vi "slider_inlet.vi"(10 "dq/dt (Flow in rate)\n[m³/s]":dbl, 11 "Slide in":refnum<vi>) -> ()   [LabVIEW 2020]
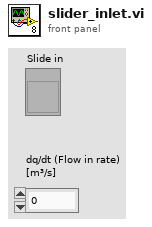
[diagram p1: front panel]
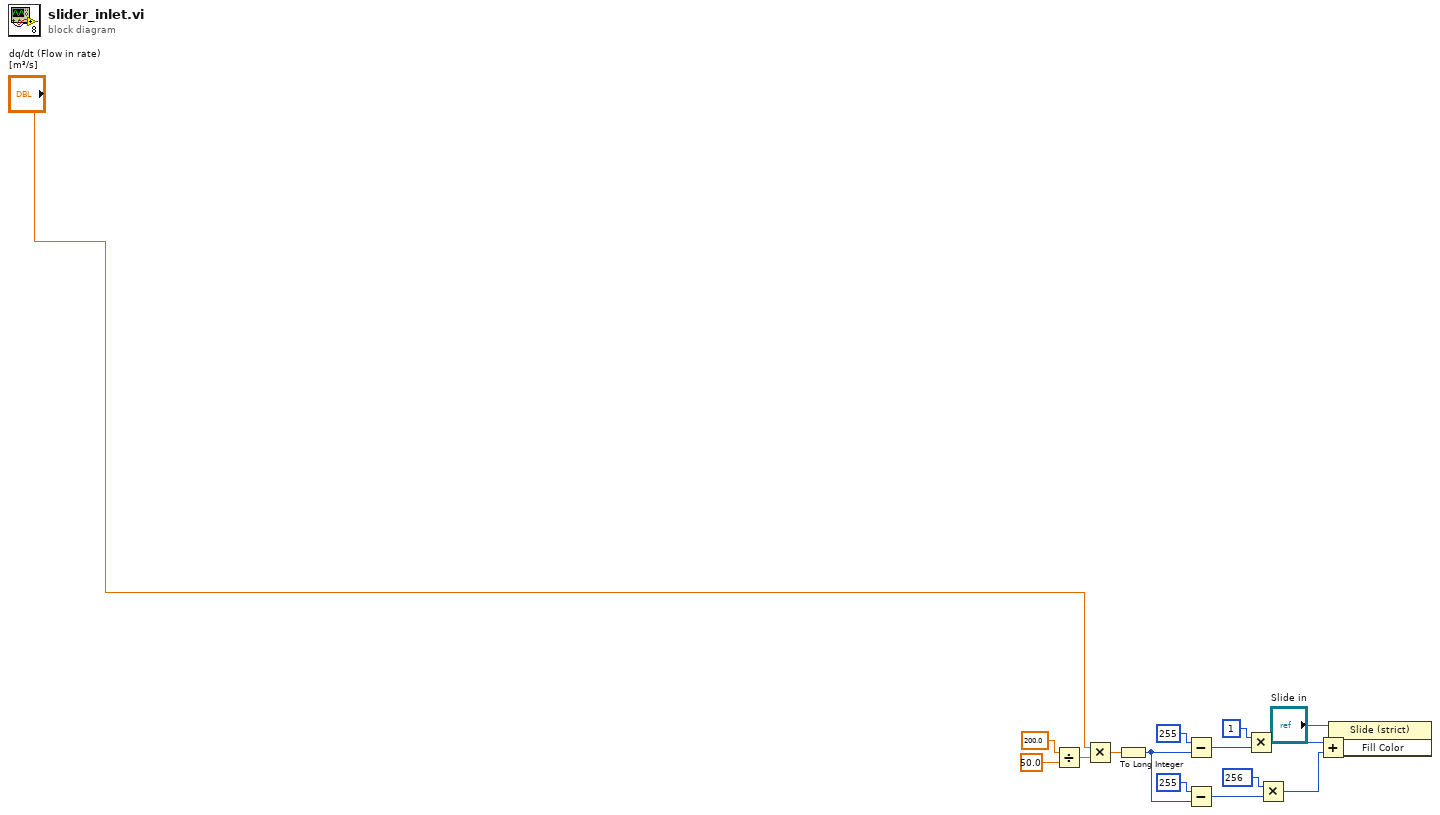
[diagram p0: block diagram]
diagram:
  n1 = Divide(x=200.0, y=50.0) -> (x/y=w13:dbl)
  n2 = Multiply(x="dq/dt (Flow in rate)\n[m³/s]", y=w13) -> (x*y=w14:dbl)
  n3 = To Long Integer(number=w14) -> (32bit integer=w9:i32)
  n4 = Subtract(x=255, y=w9) -> (x-y=w7:i32)
  n5 = Subtract(x=255, y=w9) -> (x-y=w10:i32)
  n6 = Multiply(x=1, y=w7) -> (x*y=w2:i32)
  n7 = Multiply(x=256, y=w10) -> (x*y=w3:i32)
  n8 = Add(x=w2, y=w3) -> (x+y=w15:i32)
  n9 = property on="Property Node" class="Slide (strict)"(reference="Slide in", "Fill Color"=w15) -> ()  [unwired: 1 in, 2 out]
